vi "Register Event.vi"   [LabVIEW 2019, in "Camera Engine Event.lvlib"]
uses:
  Camera Engine Event.lvlib
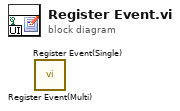
[diagram p0: block diagram]
diagram:
  n1 = call "Register Event(Multi).vi"() -> ()  [unwired: 11 in, 1 out]
  n2 = call "Register Event(Single).vi"() -> ()  [unwired: 11 in, 1 out]
